vi "SE FP Find red target.vi"(0 "Image In":T2, 1 "error in (no error)":errorcluster) -> (2 "Image Dst Out":T2, 3 "Nb Circles (Circle Detection 1)":i32, 4 "Camera Data":T1, 5 "error out":errorcluster)   [LabVIEW 2014]
doc: "This VI takes in an image and finds a round, red target. It produces the target location and size."
uses:
  <vilib>/vision/Image Controls.llb/IMAQ Image.ctl
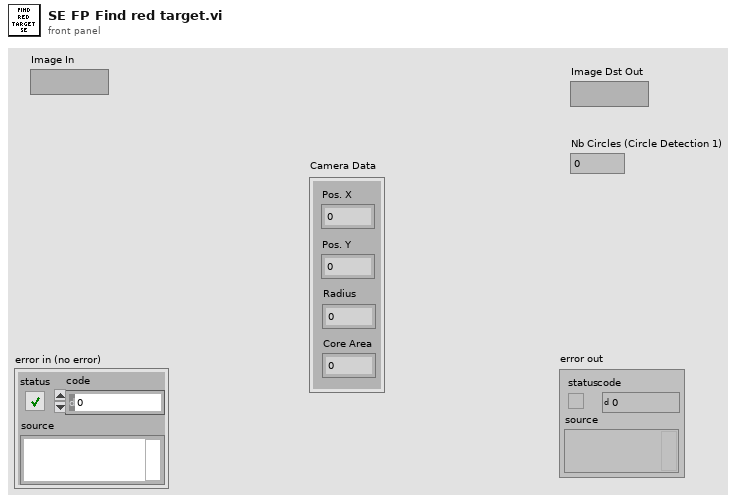
[diagram p1: front panel]
types:
  T1 = cluster{"Pos. X":i32, "Pos. Y":i32, "Radius":i32, "Core Area":i32}
  T2 = typedef "IMAQ Image.ctl" = refnum<image>
  T3 = cluster{"Pos. X":i32, "Pos. Y":i32, "Radius":i32, "Core Area":i32}[]
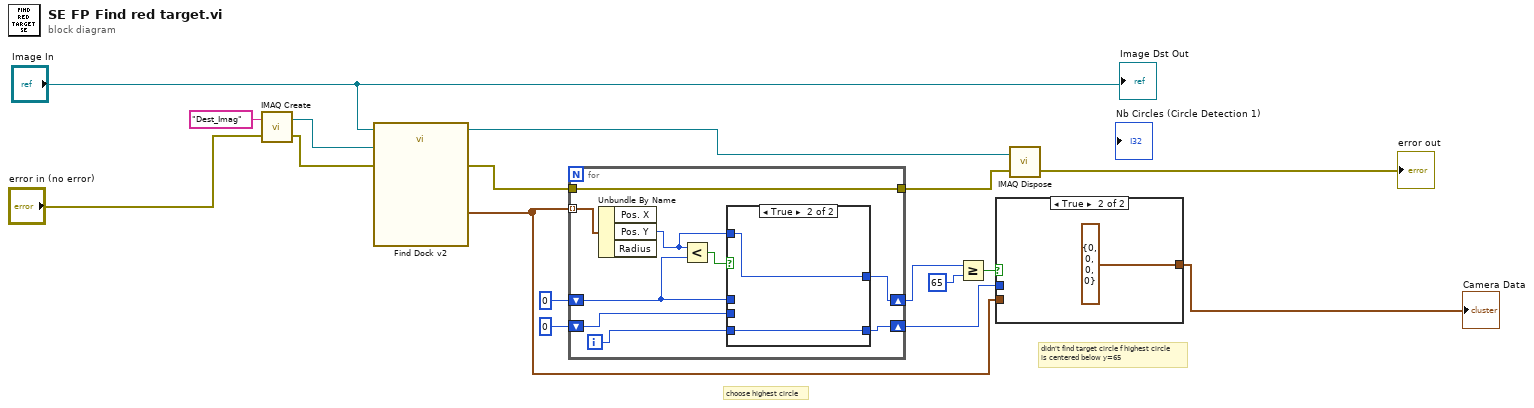
[diagram p0: block diagram]
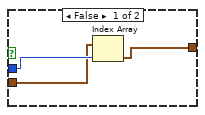
[diagram p2: hidden frame]
diagram:
  # "didn't find target circle f highest circle\nis centered below y=65"
  # "choose highest circle"
  n1 = call "IMAQ Create"("Image Name"="Dest_Imag", "error in (no error)"="error in (no error)") -> ("New Image"=w9:T2, "error out"=w10:errorcluster)  [unwired: 3 in]
  n2 = call "Find Dock v2"("Image In"="Image In", "Image Dst"=w9, "error in"=w10) -> ("Image Out"=w8:T2, "Circles Data (Circle Detection 1)"=w2:T3, "error out"=w7:errorcluster)  [unwired: 20 in, 2 out]
  n3 = for {
    tunnel: w7 -> [w26]
    tunnel: [w26] -> w14
    tunnel: w2 -> [w25] mode=indexing
    shift-right: [w22] -> w6
    shift-left: 0 -> [w21]
    shift-right: [w18] -> w3
    shift-left: 0 -> [w20]
    i -> [w19]
    n4 = Unbundle By Name(w25) -> ("Pos. Y"=w23:i32)  [unwired: 2 out]
    n5 = Less?(x=w23, y=w21) -> (x < y?=w24:bool)
    n6 = case shown="True" w24 {
      tunnel: w23 -> [_ w30]
      tunnel: [w28 w30] -> w22
      tunnel: w21 -> [w28 _]
      tunnel: w20 -> [w27 _]
      tunnel: w19 -> [_ w29]
      tunnel: [w27 w29] -> w18
      frame False {
      }
      frame True {
      }
    }
  }
  n7 = Greater Or Equal?(x=w6, y=65) -> (x >= y?=w4:bool)
  n8 = case shown="True" w4 {
    tunnel: [w31 T1 {"Pos. X"=0, "Pos. Y"=0, "Radius"=0, "Core Area"=0} ("element")] -> w1
    tunnel: w3 -> [w33 _]
    tunnel: w2 -> [w32 _]
    frame False {
      n9 = Index Array(array=w32, index=w33) -> (element=w31:T1)
    }
    frame True {
    }
  }
  "Camera Data" <- w1
  n10 = call "IMAQ Dispose"("Image"=w8, "error in (no error)"=w14) -> ("error out"=→"error out":errorcluster)  [unwired: 1 in, 3 out]
  "Image Dst Out" <- "Image In"
